vi "Parse Header.vi"(11 "HTTP Header":string) -> (3 "Headers":variant)   [LabVIEW 2013]
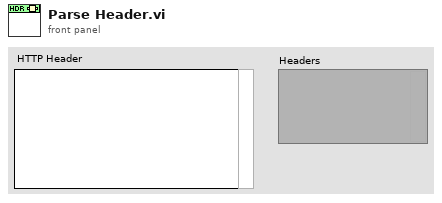
[diagram p1: front panel]
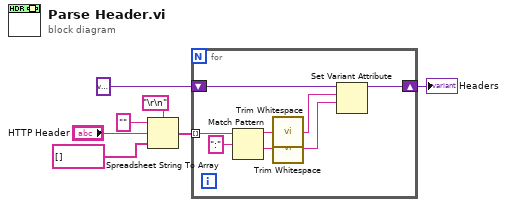
[diagram p0: block diagram]
diagram:
  n1 = Spreadsheet String To Array(delimiter (Tab)="\r\n" ("format string"), format string="", spreadsheet string="HTTP Header", array type (2D Dbl)=string[] []) -> (array=w3:string[])
  n2 = for {
    tunnel: w3 -> [w15] mode=indexing
    shift-right: [w8] -> w1
    shift-left: variant ("variant") -> [w9]
    n3 = Match Pattern(string=w15, regular expression=":") -> (before substring=w13:string, after substring=w12:string)  [unwired: 1 in, 2 out]
    n4 = call <vilib>:"Trim Whitespace.vi"("string"=w13) -> ("trimmed string"=w11:string)  [unwired: 1 in]
    n5 = call <vilib>:"Trim Whitespace.vi"("string"=w12) -> ("trimmed string"=w10:string)  [unwired: 1 in]
    n6 = Set Variant Attribute(Variant=w9, name=w11, value=w10) -> (Variant out=w8:variant)  [unwired: 1 in, 2 out]
  }
  "Headers" <- w1
